vi "GetVision.vi"(7 "Robot_H (deg)":dbl) -> (4 "LimeLight Raw Z (in)":dbl, 6 "LimeLight Raw X (in)":dbl, 8 "LimeLight Distance to Target (in)":dbl, 10 "LimeLight Raw Horizontal Offset (deg)":dbl, 15 "LimeLight Heading to Target (deg)":dbl)   [LabVIEW 2019]
doc: "This VI reads the raw data from the LimeLight pipeline and runs several validity checks."
uses:
  <vilib>/Rock Robotics/Network Tables/NT Read Numeric Array.vi
  <vilib>/Rock Robotics/Network Tables/NT Read Number.vi
  dsdata.vi
  sensors.vi
panel:
  in  "Maximum Pointing Error (deg)":dbl=15.0
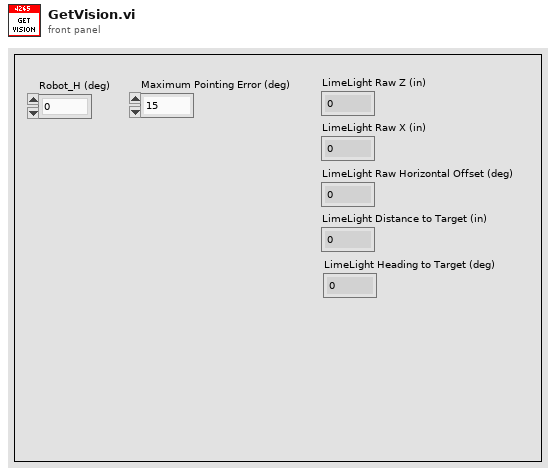
[diagram p1: front panel]
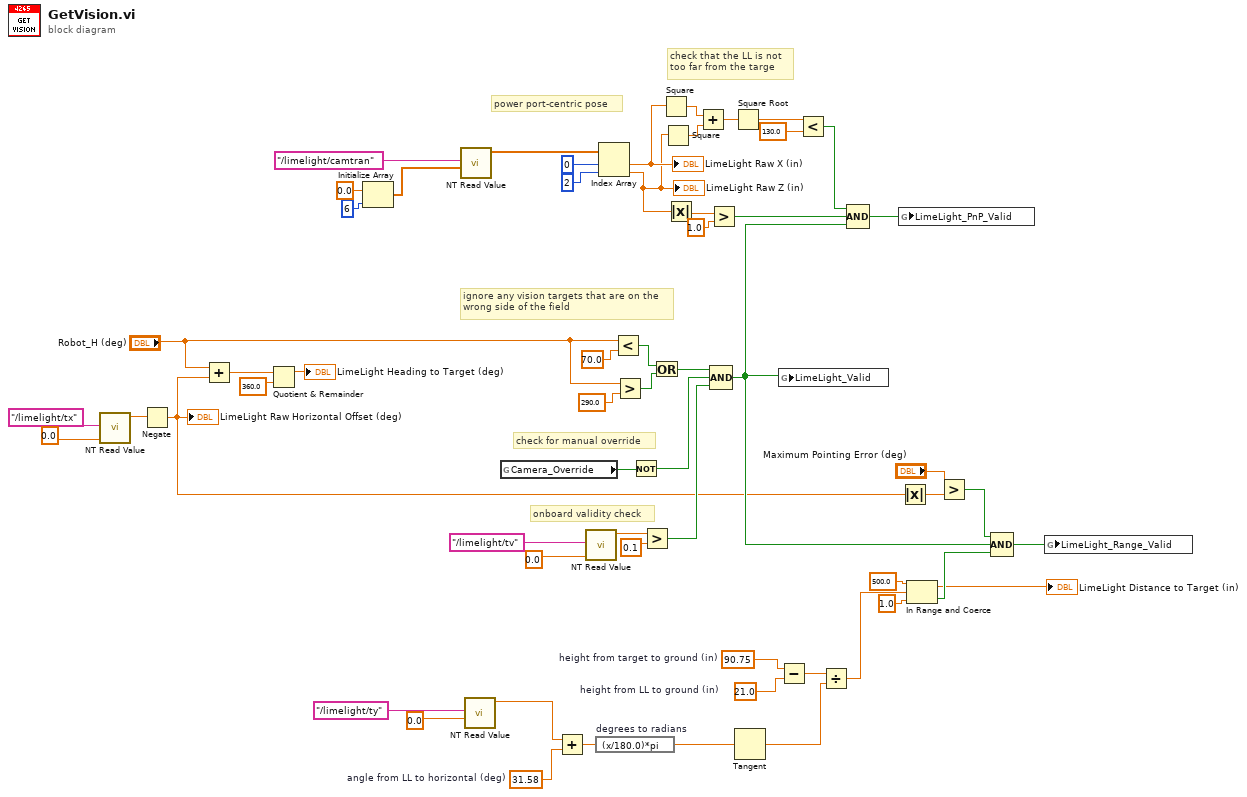
[diagram p0: block diagram]
diagram:
  w20 = 31.58  # angle from LL to horizontal (deg)
  w25 = 21.0  # height from LL to ground (in)
  w26 = 90.75  # height from target to ground (in)
  # "check for manual override"
  # "onboard validity check"
  # "check that the LL is not\ntoo far from the targe"
  # "power port-centric pose"
  # "ignore any vision targets that are on the\nwrong side of the field"
  n1 = call-poly <vilib>:"NT Read Value.vi"("Default Value"=0.0, "Name"="/limelight/tx") -> ("Numeric"=w27:dbl)  [unwired: 8 in, 1 out]
  n2 = Negate(x=w27) -> (-x=w2:dbl)
  "LimeLight Raw Horizontal Offset (deg)" <- w2
  n3 = Add(x="Robot_H (deg)", y=w2) -> (x+y=w15:dbl)
  n4 = Quotient & Remainder(x=w15, y=360.0) -> (x-y*floor(x/y)=→"LimeLight Heading to Target (deg)":dbl)  [unwired: 1 out]
  n5 = Initialize Array(0.0 ("element"), 6 ("dimension size")) -> (w56:dbl[])
  n6 = call-poly <vilib>:"NT Read Value.vi"("Default Value"=w56, "Name"="/limelight/camtran") -> ("Numeric Array"=w53:dbl[])  [unwired: 8 in, 1 out]
  n7 = call-poly <vilib>:"NT Read Value.vi"("Default Value"=0.0, "Name"="/limelight/ty") -> ("Numeric"=w21:dbl)  [unwired: 8 in, 1 out]
  n8 = global read "dsdata.vi" "Camera_Override"() -> (w45:bool)
  n9 = Add(x=w21, y=w20) -> (x+y=w19:dbl)
  n10 = call-poly <vilib>:"NT Read Value.vi"("Default Value"=0.0, "Name"="/limelight/tv") -> ("Numeric"=w48:dbl)  [unwired: 8 in, 1 out]
  n11 = expression code="(x/180.0)*pi" "degrees to radians"(w19) -> (w18:dbl)
  n12 = Index Array(array=w53, index #1=0 ("index"), index #2=2 ("index")) -> (element #1=w32:dbl, element #2=w31:dbl)
  "LimeLight Raw X (in)" <- w32
  "LimeLight Raw Z (in)" <- w31
  n13 = Less?(x="Robot_H (deg)", y=70.0) -> (x < y?=w41:bool)
  n14 = Greater?(x="Robot_H (deg)", y=290.0) -> (0:w42:bool)
  n15 = Not(x=w45) -> (.not. x?=w38:bool)
  n16 = Greater?(x=w48, y=0.1) -> (0:w46:bool)
  n17 = Or(x=w41, y=w42) -> (x .or. y?=w39:bool)
  n18 = Square(x=w32) -> (x^2=w37:dbl)
  n19 = Square(x=w31) -> (x^2=w36:dbl)
  n20 = Absolute Value(x=w31) -> (abs(x)=w52:dbl)
  n21 = Add(x=w37, y=w36) -> (x+y=w35:dbl)
  n22 = Greater?(x=w52, y=1.0) -> (0:w40:bool)
  n23 = Compound Arithmetic op=AND(w39, w38, w46) -> (w16:bool)
  n24 = Square Root(x=w35) -> (sqrt(x)=w34:dbl)
  n25 = Tangent(1:w18) -> (0:w17:dbl)
  n26 = global write "sensors.vi" "LimeLight_Valid"(w16) -> ()
  n27 = Subtract(x=w26, y=w25) -> (x-y=w24:dbl)
  n28 = Less?(x=w34, y=130.0) -> (x < y?=w30:bool)
  n29 = Divide(x=w24, y=w17) -> (x/y=w9:dbl)
  n30 = Compound Arithmetic op=AND(w30, w40, w16) -> (w11:bool)
  n31 = global write "sensors.vi" "LimeLight_PnP_Valid"(w11) -> ()
  n32 = Absolute Value(x=w2) -> (abs(x)=w4:dbl)
  n33 = In Range and Coerce(upper limit=500.0, x=w9, lower limit=1.0) -> (coerced(x)=→"LimeLight Distance to Target (in)":dbl, In Range?=w6:bool)
  n34 = Greater?(x="Maximum Pointing Error (deg)", y=w4) -> (0:w1:bool)
  n35 = Compound Arithmetic op=AND(w1, w16, w6) -> (w10:bool)
  n36 = global write "sensors.vi" "LimeLight_Range_Valid"(w10) -> ()
